vi "WAPIAerOpen.vi"(8 "error in (no error)":errorcluster, 11 "board":i16) -> (0 "error out":errorcluster)   [LabVIEW 2009]
uses:
  win50032.dll
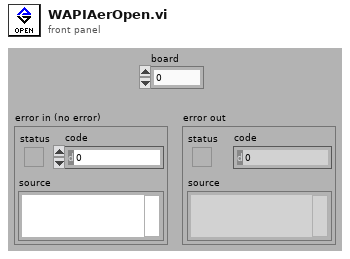
[diagram p1: front panel]
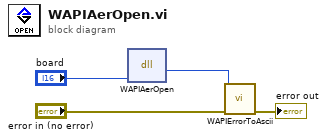
[diagram p0: block diagram]
diagram:
  n1 = dll-call lib="Win50032.dll" fn="WAPIAerOpen"("board"="board") -> ("return type"=w4:u32)  [unwired: 4 in, 2 out]
  n2 = call "WAPIErrorToAscii.vi"("error in (no error)"="error in (no error)", "error"=w4) -> ("error out"=→"error out":errorcluster)  [unwired: 8 in, 1 out]
